vi "Write Results.vi"(8 "error in (no error)":errorcluster, 10 "Results":refnum<class "Acquired Result.lvclass">[](array[class]), 11 "Process Controller in":refnum<class "Process Controller.lvclass">) -> (0 "error out":errorcluster, 3 "Process Controller out":refnum<class "Process Controller.lvclass">)   [LabVIEW 2021, in "Process Controller.lvclass"]
uses:
  Process Controller.lvclass
  Process Controller.lvclass/Process Controller.ctl
  NHMFL_Core/Libraries/Instruments/Results/Acquired Result/Acquired Result.lvclass
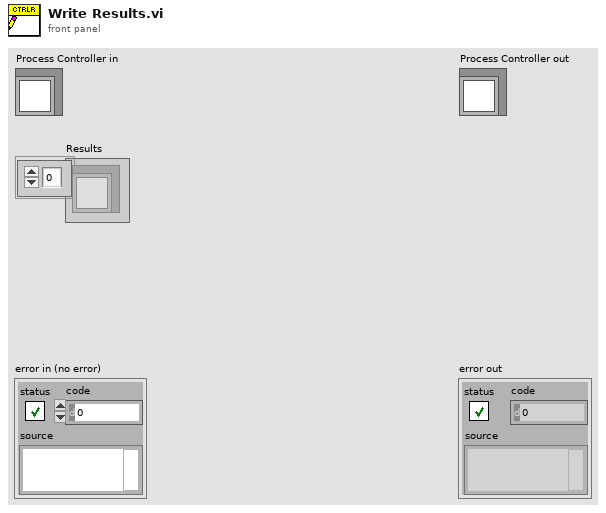
[diagram p1: front panel]
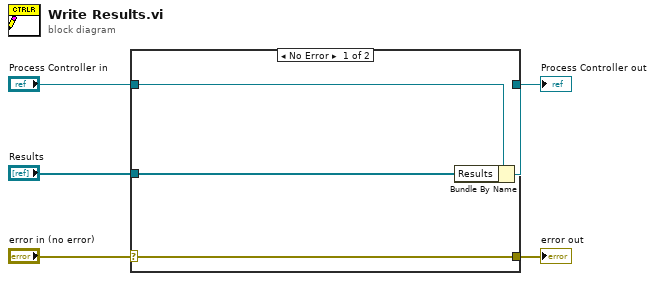
[diagram p0: block diagram]
diagram:
  n1 = case shown="No Error" "error in (no error)" {
    selector: "error in (no error)" -> [w9 w10]
    tunnel: [w9 w10] -> w4
    tunnel: [w7 w11] -> w2
    tunnel: "Process Controller in" -> [w8 w11]
    tunnel: "Results" -> [w6 _]
    frame No Error {
      n2 = Bundle By Name(cluster=w8, "Results"=w6) -> (w7:refnum<class "Process Controller.lvclass">)
    }
    frame Error {
    }
  }
  "error out" <- w4
  "Process Controller out" <- w2
